vi "Temperature Monitor.vi"() -> ()   [LabVIEW 2014]
doc: "이 VI는 LabVIEW Core I 교육 과정의 연습문제에 대한 해답입니다.\n\n이 VI는 While 루프와 시프트 레지스터를 사용하여 데이터의 평균을 구합니다. 하드웨어는 필요하지 않습니다."
panel:
  in  "정지 버튼":bool
  out "온도 히스토리":dbl(graph)
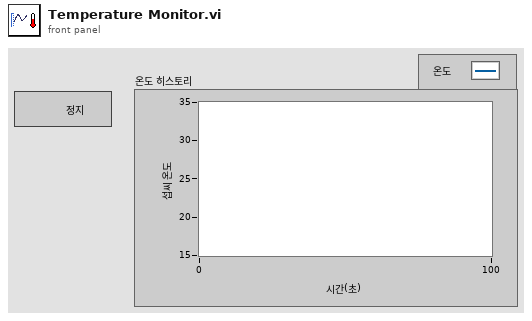
[diagram p1: front panel]
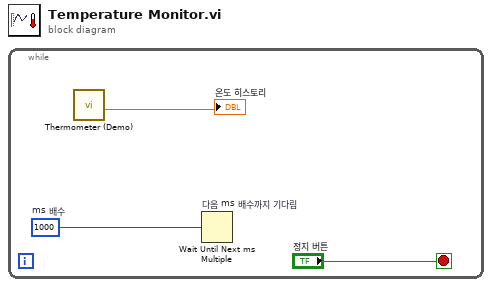
[diagram p0: block diagram]
diagram:
  n1 = while {
    stop <- "정지 버튼" stop-if-true
    w3 = u32 1000  # ms 배수
    n2 = call "Thermometer (Demo).vi"() -> ("온도 값"=→"온도 히스토리":dbl)  [unwired: 11 in]
    n3 = Wait Until Next ms Multiple "다음 ms 배수까지 기다림"(millisecond multiple=w3) -> ()  [unwired: 1 out]
  }
